vi "GetRectAndLineIntersection.vi"(4 "y2 In":i32, 6 "x2 In":i32, 8 "No Error":errorcluster, 9 "y1 In":i32, 10 "x1 In":i32, 11 "Rect":T1) -> (0 "Error Out":errorcluster, 1 "y1 Out":i32, 2 "x1 Out":i32, 3 "Intersect?":bool, 5 "y2 Out":i32, 7 "x2 Out":i32)   [LabVIEW 2026, in "SDL3.lvlib" / "Rect.lvlib"]
doc: "<B>Summary</B>\nCalculate the intersection of a rectangle and line segment.\n\n<B>Remarks</B>\nThis function is used to clip a line segment to a rectangle. A line segment contained entirely within the rectangle or that does not intersect will remain unchanged. A line segment that crosses the rectangle at either or both ends will be clipped to the boundary of the rectangle and the new coordinates saved in X1, Y1, X2, and/or Y2 as necessary."
uses:
  Rect.lvlib
  Rect--cluster.ctl
  Lib/SDL3.dll
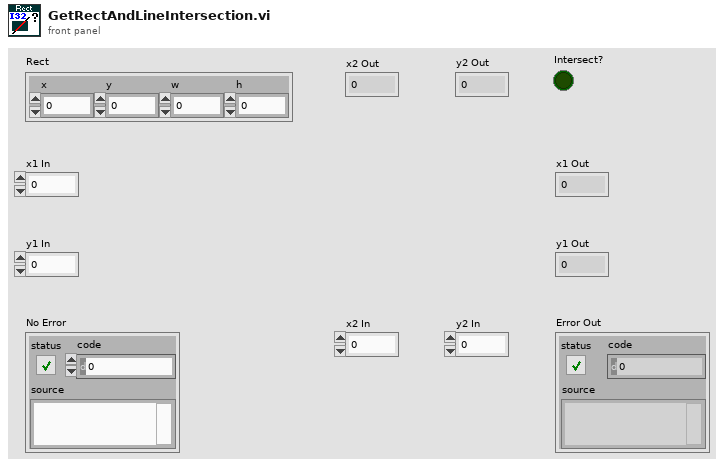
[diagram p1: front panel]
types:
  T1 = typedef "SDL3.lvlib/Rect.lvlib/Rect--cluster.ctl" = cluster{"x":i32, "y":i32, "w":i32, "h":i32}
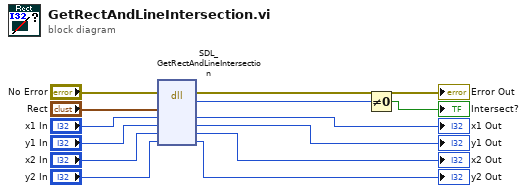
[diagram p0: block diagram]
diagram:
  n1 = dll-call lib="C:/Users/saukko/Dev/LV-SDL3/Sources/SDL3/Lib/SDL3.*" fn="SDL_GetRectAndLineIntersection"(error in="No Error", "rect"="Rect", "X1"="x1 In", "Y1"="y1 In", "X2"="x2 In", "Y2"="y2 In") -> (error out=→"Error Out":errorcluster, "return type"=w11:i32, "X1"=→"x1 Out":i32, "Y1"=→"y1 Out":i32, "X2"=→"x2 Out":i32, "Y2"=→"y2 Out":i32)  [unwired: 3 in, 1 out]
  n2 = Not Equal To 0?(x=w11) -> (x != 0?=→"Intersect?":bool)
